vi "CorridorBeam.vi"(0 "error in (no error)":errorcluster) -> (1 "error out":errorcluster, 2 "return type":i16)   [LabVIEW 2013]
doc: "Use this template to build a VI to use as a subVI."
uses:
  704IO.dll
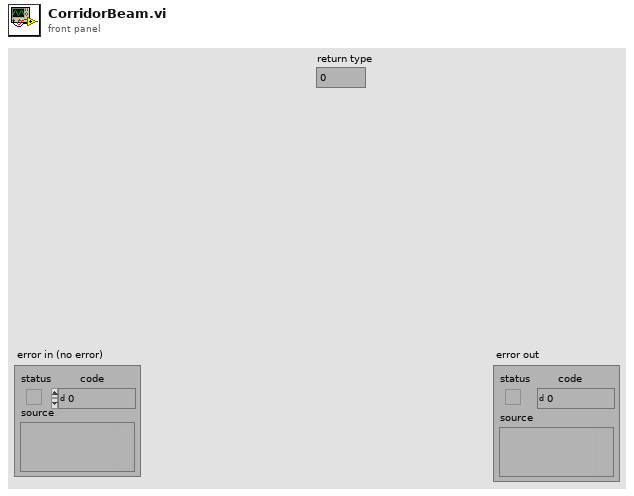
[diagram p1: front panel]
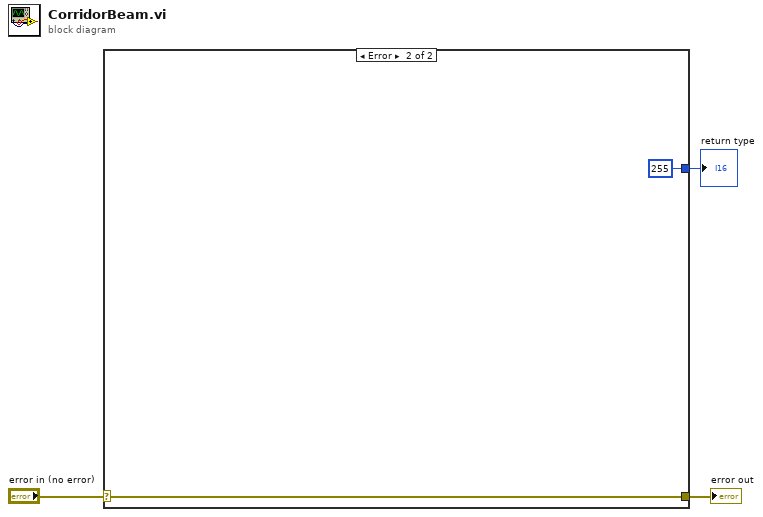
[diagram p0: block diagram]
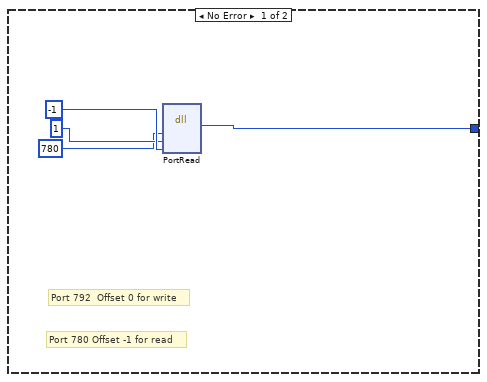
[diagram p2: hidden frame]
diagram:
  n1 = case shown="Error" "error in (no error)" {
    selector: "error in (no error)" -> [_ w9]
    tunnel: [_ w9] -> w2
    tunnel: [w4 i16 255 ("return type")] -> w1
    frame No Error {
      # "Port 780 Offset -1 for read"
      # "Port 792  Offset 0 for write"
      n2 = dll-call lib="C:/Users/Radu Darie/Documents/GitHub/ParkinsonsCorridor/704IO.dll" fn="PortRead"("Port"=i16 780, "Rack"=i16 1, "Offset"=i16 -1) -> ("return type"=w4:i16)  [unwired: 6 in, 2 out]
    }
    frame Error {
    }
  }
  "error out" <- w2
  "return type" <- w1
